vi "queue_same_name.vi"() -> ()   [LabVIEW 2021]
panel:
  out "element 2":i32
  out "element":i32
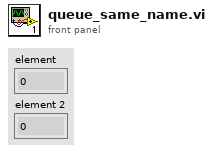
[diagram p1: front panel]
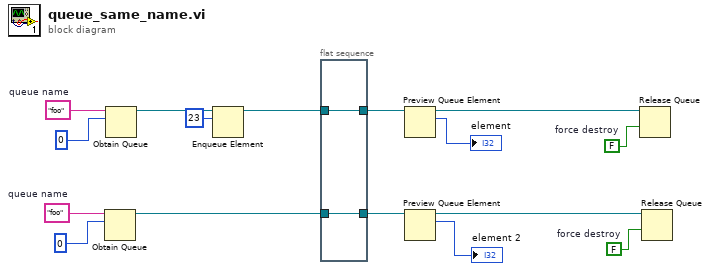
[diagram p0: block diagram]
diagram:
  w2 = FALSE  # force destroy
  w3 = FALSE  # force destroy
  w9 = "foo"  # queue name
  w16 = "foo"  # queue name
  n1 = Obtain Queue(name (unnamed)=w9, element data type=0) -> (queue out=w8:refnum<queue>)  [unwired: 3 in, 2 out]
  n2 = Obtain Queue(name (unnamed)=w16, element data type=0) -> (queue out=w14:refnum<queue>)  [unwired: 3 in, 2 out]
  n3 = Enqueue Element(queue=w14, element=23) -> (queue out=w13:refnum<queue>)  [unwired: 2 in, 2 out]
  n4 = flat-sequence {
    tunnel: w13 -> [w18]
    tunnel: [w18] -> w12
    tunnel: [w17] -> w7
    tunnel: w8 -> [w17]
    frame #0 {
    }
  }
  n5 = Preview Queue Element(queue=w12) -> (queue out=w4:refnum<queue>, element=→"element":i32)  [unwired: 2 in, 2 out]
  n6 = Preview Queue Element(queue=w7) -> (queue out=w1:refnum<queue>, element=→"element 2":i32)  [unwired: 2 in, 2 out]
  n7 = Release Queue(queue=w4, force destroy? (F)=w3) -> ()  [unwired: 1 in, 3 out]
  n8 = Release Queue(queue=w1, force destroy? (F)=w2) -> ()  [unwired: 1 in, 3 out]
